vi "Name To Index.vi"(5 "Name":string) -> (2 "Index":i32)   [LabVIEW 2019, in "Setting Database.lvclass"]
uses:
  Setting Database.lvclass
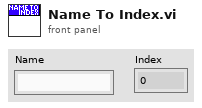
[diagram p1: front panel]
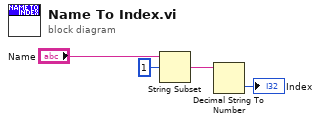
[diagram p0: block diagram]
diagram:
  n1 = String Subset(string="Name", offset (0)=1) -> (substring=w2:string)  [unwired: 1 in]
  n2 = Decimal String To Number(string=w2) -> (number=→"Index":i32)  [unwired: 2 in, 1 out]
